vi "VisionExecute.v.vi"(8 "error in (no error)":errorcluster) -> (0 "error out":errorcluster)   [LabVIEW 2023]
uses:
  <vilib>/Rock Robotics/WPI/ThirdParty/PhotonVisionLib/Enum/PhotonPoseStrategy_ENUM.ctl
  <vilib>/Rock Robotics/WPI/ThirdParty/JAS_Junk/TrajLib/TypeDef/POSE2D.ctl
  <vilib>/Rock Robotics/WPI/ThirdParty/JAS_Junk/TrajLib/TypeDef/TRANSLATION2D.ctl
  <vilib>/Rock Robotics/WPI/ThirdParty/JAS_Junk/TrajLib/TypeDef/ROTATION2D.ctl
  <vilib>/Rock Robotics/WPI/ThirdParty/JAS_Junk/TrajLib/VI/AprilTagFieldLayout_New2025.vi
  <vilib>/Rock Robotics/WPI/ThirdParty/JAS_Junk/TrajLib/VI/Util_GetTime_U32.vi
  <vilib>/Rock Robotics/WPI/ThirdParty/PhotonVisionLib/SubVI/PhotonPipelineResult_Unpack.vi
  <vilib>/Rock Robotics/WPI/ThirdParty/PhotonVisionLib/SubVI/PhotonPipelineResult_GetTargetCount.vi
  <vilib>/Rock Robotics/WPI/ThirdParty/PhotonVisionLib/SubVI/PhotonPipelineResult_GetMetadata.vi
  <vilib>/Rock Robotics/WPI/ThirdParty/PhotonVisionLib/SubVI/PhotonPipelineMetadata_GetAll.vi
  <vilib>/Rock Robotics/WPI/ThirdParty/JAS_Junk/TrajLib/VI/Transform3d_Equals.vi
  <vilib>/Rock Robotics/WPI/ThirdParty/PhotonVisionLib/SubVI/PhotonPoseEstimator_SetCamera.vi
  <vilib>/Rock Robotics/WPI/ThirdParty/PhotonVisionLib/SubVI/PhotonPoseEstimator_SetPrimaryStategy.vi
  <vilib>/Rock Robotics/WPI/ThirdParty/PhotonVisionLib/SubVI/PhotonPoseEstimator_SetMultiTagFallbackStrategy.vi
  <vilib>/Rock Robotics/WPI/ThirdParty/PhotonVisionLib/SubVI/PhotonPoseEstimator_SetHighestAmbiguity.vi
  <vilib>/Rock Robotics/WPI/ThirdParty/PhotonVisionLib/SubVI/PhotonPoseEstimator_SetRobotToCameraTransform.vi
  <vilib>/Rock Robotics/WPI/ThirdParty/PhotonVisionLib/SubVI/PhotonPoseEstimator_New.vi
  <vilib>/Rock Robotics/WPI/ThirdParty/PhotonVisionLib/SubVI/PhotonPoseEstimator_SetLastPose.vi
  <vilib>/Rock Robotics/WPI/ThirdParty/PhotonVisionLib/SubVI/PhotonPoseEstimator_Update_PipeResult.vi
  <vilib>/Rock Robotics/WPI/ThirdParty/PhotonVisionLib/SubVI/PhotonPoseEstimator_SetReferencePose.vi
  <vilib>/Rock Robotics/WPI/ThirdParty/PhotonVisionLib/SubVI/PhotonEstimatedRobotPose_GetAll.vi
  <vilib>/Rock Robotics/WPI/ThirdParty/JAS_Junk/TrajLib/VI/Pose3d_ToPose2d.vi
  <vilib>/Rock Robotics/WPI/ThirdParty/JAS_Junk/TrajLib/VI/Quaternion_New.vi
  <vilib>/Rock Robotics/WPI/ThirdParty/JAS_Junk/TrajLib/Conv_Deg_Radians.vi
  <vilib>/Rock Robotics/WPI/ThirdParty/JAS_Junk/TrajLib/VI/TimeInterpDouble_New.vi
  <vilib>/Rock Robotics/WPI/ThirdParty/JAS_Junk/TrajLib/VI/TimeInterpDouble_AddSample.vi
  <vilib>/Rock Robotics/WPI/ThirdParty/JAS_Junk/TrajLib/VI/TimeInterpDouble_GetSample.vi
  <vilib>/Rock Robotics/WPI/ThirdParty/JAS_Junk/TrajLib/VI/TimeInterpDouble_SetMaxTime.vi
  <vilib>/Rock Robotics/WPI/ThirdParty/JAS_Junk/TrajLib/Twist2d_GetAll.vi
  <vilib>/Rock Robotics/WPI/ThirdParty/JAS_Junk/TrajLib/Twist2d_Create.vi
  <vilib>/Rock Robotics/WPI/ThirdParty/JAS_Junk/TrajLib/VI/AprilTagFieldLayout_New.vi
  <vilib>/Rock Robotics/WPI/ThirdParty/JAS_Junk/TrajLib/VI/Pose3d_New_Trans3dRot3d.vi
  <vilib>/Rock Robotics/WPI/ThirdParty/JAS_Junk/TrajLib/VI/Rotation3d_Create_Quaternion.vi
  <vilib>/Rock Robotics/WPI/ThirdParty/JAS_Junk/TrajLib/VI/AprilTag_New.vi
  <vilib>/Rock Robotics/WPI/ThirdParty/JAS_Junk/TrajLib/Timer_New.vi
  <vilib>/Rock Robotics/WPI/ThirdParty/PhotonVisionLib/SubVI/Packet_decode_ByteI8.vi
  <vilib>/Rock Robotics/WPI/ThirdParty/PhotonVisionLib/SubVI/PhotonTrackedTarget_Unpack.vi
  <vilib>/Rock Robotics/WPI/ThirdParty/PhotonVisionLib/SubVI/PhotonMultiTargetPNPResult_unpack.vi
  <vilib>/Rock Robotics/WPI/ThirdParty/PhotonVisionLib/SubVI/PhotonPipelineMetadata_Unpack.vi
  <vilib>/Rock Robotics/WPI/ThirdParty/PhotonVisionLib/SubVI/PhotonPipelineResult_New.vi
  <vilib>/Rock Robotics/WPI/ThirdParty/JAS_Junk/TrajLib/VI/Transform3d_GetTranslation3d.vi
  <vilib>/Rock Robotics/WPI/ThirdParty/JAS_Junk/TrajLib/VI/Transform3d_GetRotation3d.vi
  <vilib>/Rock Robotics/WPI/ThirdParty/JAS_Junk/TrajLib/VI/Rotation3d_Equals.vi
  <vilib>/Rock Robotics/WPI/ThirdParty/JAS_Junk/TrajLib/VI/Translation3d_Equals.vi
  <vilib>/Rock Robotics/WPI/ThirdParty/PhotonVisionLib/SubVI/PhotonTargetModel_New_AprilTag36H11.vi
  <vilib>/Rock Robotics/WPI/ThirdParty/PhotonVisionLib/SubVI/PhotonPoseEstimator_Update_All.vi
  <vilib>/Rock Robotics/WPI/ThirdParty/JAS_Junk/TrajLib/VI/Pose3d_getTranslation3d.vi
  <vilib>/Rock Robotics/WPI/ThirdParty/JAS_Junk/TrajLib/VI/Pose3d_getRotation3d.vi
  <vilib>/Rock Robotics/WPI/ThirdParty/JAS_Junk/TrajLib/VI/Translation3d_ToTranslation2d.vi
  <vilib>/Rock Robotics/WPI/ThirdParty/JAS_Junk/TrajLib/VI/Rotation3d_ToRotation2d.vi
  <vilib>/Rock Robotics/WPI/ThirdParty/JAS_Junk/TrajLib/Pose2d_New_TRRO.vi
  <vilib>/Rock Robotics/WPI/ThirdParty/JAS_Junk/TrajLib/VI/TimeInterpDouble_CleanUp.vi
  <vilib>/Rock Robotics/WPI/ThirdParty/JAS_Junk/TrajLib/MathUtil_Interpolate.vi
  <vilib>/Rock Robotics/WPI/ThirdParty/JAS_Junk/TrajLib/VI/AprilTag_GetAll.vi
  <vilib>/Rock Robotics/WPI/ThirdParty/JAS_Junk/TrajLib/VI/Quaternion_Normalize.vi
  <vilib>/Rock Robotics/WPI/ThirdParty/PhotonVisionLib/SubVI/Packet_decode_Flt64.vi
  <vilib>/Rock Robotics/WPI/ThirdParty/PhotonVisionLib/SubVI/TargetCorner_New.vi
  <vilib>/Rock Robotics/WPI/ThirdParty/PhotonVisionLib/SubVI/Packet_decode_Int32.vi
  <vilib>/Rock Robotics/WPI/ThirdParty/PhotonVisionLib/SubVI/Packet_decode_Transform3d.vi
  <vilib>/Rock Robotics/WPI/ThirdParty/PhotonVisionLib/SubVI/Packet_decode_Flt32.vi
  <vilib>/Rock Robotics/WPI/ThirdParty/PhotonVisionLib/SubVI/Packet_decode_TargetCornerArray.vi
  <vilib>/Rock Robotics/WPI/ThirdParty/PhotonVisionLib/SubVI/Packet_decode_Boolean.vi
  <vilib>/Rock Robotics/WPI/ThirdParty/PhotonVisionLib/SubVI/PhotonPNPResult_unpack.vi
  <vilib>/Rock Robotics/WPI/ThirdParty/PhotonVisionLib/SubVI/PhotonMultiTargetPNPResult_New.vi
  <vilib>/Rock Robotics/WPI/ThirdParty/PhotonVisionLib/SubVI/Packet_decode_Int16.vi
  <vilib>/Rock Robotics/WPI/ThirdParty/PhotonVisionLib/SubVI/Packet_decode_Int64.vi
  <vilib>/Rock Robotics/WPI/ThirdParty/JAS_Junk/TrajLib/VI/Rotation3d_GetQuaterion.vi
  <vilib>/Rock Robotics/WPI/ThirdParty/JAS_Junk/TrajLib/VI/Quaternion_Equals.vi
  <vilib>/Rock Robotics/WPI/ThirdParty/PhotonVisionLib/SubVI/PhotonTargetModel_New_RectPlanar.vi
  <vilib>/Rock Robotics/WPI/ThirdParty/PhotonVisionLib/SubVI/PhotonPoseEstimator_GetEmptyPose.vi
  <vilib>/Rock Robotics/WPI/ThirdParty/PhotonVisionLib/SubVI/PhotonPoseEstimator_lowestAmbiguityStrategy.vi
  <vilib>/Rock Robotics/WPI/ThirdParty/PhotonVisionLib/SubVI/PhotonPoseEstimator_closestToCameraHeightStrategy.vi
  <vilib>/Rock Robotics/WPI/ThirdParty/PhotonVisionLib/SubVI/PhotonPoseEstimator_closestToReferencePoseStrategy.vi
  <vilib>/Rock Robotics/WPI/ThirdParty/PhotonVisionLib/SubVI/PhotonPoseEstimator_GetReferencePose.vi
  <vilib>/Rock Robotics/WPI/ThirdParty/PhotonVisionLib/SubVI/PhotonPoseEstimator_GetLastPose.vi
  <vilib>/Rock Robotics/WPI/ThirdParty/PhotonVisionLib/SubVI/PhotonPoseEstimator_averageBestTargetsStrategy.vi
  <vilib>/Rock Robotics/WPI/ThirdParty/PhotonVisionLib/SubVI/PhotonPoseEstimator_multiTagOnCoprocStrategy.vi
  <vilib>/Rock Robotics/WPI/ThirdParty/PhotonVisionLib/SubVI/PhotonPipelineResult_GetTimeStampSecs.vi
  <vilib>/Rock Robotics/WPI/ThirdParty/JAS_Junk/TrajLib/Translation2d_Create.vi
  <vilib>/Rock Robotics/WPI/ThirdParty/JAS_Junk/TrajLib/Rotation2d_CreateAngle.vi
  <vilib>/Rock Robotics/WPI/ThirdParty/JAS_Junk/TrajLib/VI/Rotation3d_GetXYZ.vi
  <vilib>/Rock Robotics/WPI/ThirdParty/JAS_Junk/TrajLib/MathUtil_Clamp.vi
  <vilib>/Rock Robotics/WPI/ThirdParty/JAS_Junk/TrajLib/VI/Quaternion_New_Default.vi
  <vilib>/Rock Robotics/WPI/ThirdParty/PhotonVisionLib/SubVI/PhotonPNPResult_New.vi
  <vilib>/Rock Robotics/WPI/ThirdParty/JAS_Junk/TrajLib/VI/Quaternion_Get_Vect.vi
  <vilib>/Rock Robotics/WPI/ThirdParty/JAS_Junk/TrajLib/VI/Quaternion_Get_W.vi
  <vilib>/Rock Robotics/WPI/ThirdParty/PhotonVisionLib/SubVI/PhotonTargetModel_New.vi
  <vilib>/Rock Robotics/WPI/ThirdParty/JAS_Junk/TrajLib/VI/Rotation3d_Create_AxisAngle.vi
  <vilib>/Rock Robotics/WPI/ThirdParty/JAS_Junk/TrajLib/VI/Pose3d_New.vi
  <vilib>/Rock Robotics/WPI/ThirdParty/PhotonVisionLib/SubVI/PhotonPipelineResult_HasTargets.vi
  <vilib>/Rock Robotics/WPI/ThirdParty/PhotonVisionLib/SubVI/PhotonPipelineResult_GetTargets.vi
  <vilib>/Rock Robotics/WPI/ThirdParty/PhotonVisionLib/SubVI/PhotonTrackedTarget_GetPoseAmbiguity.vi
  <vilib>/Rock Robotics/WPI/ThirdParty/PhotonVisionLib/SubVI/PhotonTrackedTarget_GetFiducialId.vi
  <vilib>/Rock Robotics/WPI/ThirdParty/PhotonVisionLib/SubVI/PhotonPoseEstimator_GetFieldTags.vi
  <vilib>/Rock Robotics/WPI/ThirdParty/JAS_Junk/TrajLib/VI/AprilTagFieldLayout_GetTagPose.vi
  <vilib>/Rock Robotics/WPI/ThirdParty/JAS_Junk/TrajLib/VI/Pose3d_TransformBy.vi
  <vilib>/Rock Robotics/WPI/ThirdParty/PhotonVisionLib/SubVI/PhotonTrackedTarget_GetBestCameraToTarget.vi
  <vilib>/Rock Robotics/WPI/ThirdParty/JAS_Junk/TrajLib/VI/Transform3d_Inverse.vi
  <vilib>/Rock Robotics/WPI/ThirdParty/PhotonVisionLib/SubVI/PhotonPoseEstimator_GetRobotToCameraTransform.vi
  <vilib>/Rock Robotics/WPI/ThirdParty/PhotonVisionLib/SubVI/PhotonPoseEstimator_GetHighestAmbiguity.vi
  <vilib>/Rock Robotics/WPI/ThirdParty/PhotonVisionLib/SubVI/PhotonEstimatedRobotPose_New.vi
  <vilib>/Rock Robotics/WPI/ThirdParty/PhotonVisionLib/SubVI/PhotonPoseEstimator_closestToCameraHeightStrategy_calc.vi
  <vilib>/Rock Robotics/WPI/ThirdParty/PhotonVisionLib/SubVI/PhotonTrackedTarget_GetAltCameraToTarget.vi
  <vilib>/Rock Robotics/WPI/ThirdParty/PhotonVisionLib/SubVI/PhotonPoseEstimator_closestToReferencePoseStrategy_calc.vi
  <vilib>/Rock Robotics/WPI/ThirdParty/PhotonVisionLib/SubVI/PhotonPoseEstimator_averageBestTargetsStrategy_calc.vi
  <vilib>/Rock Robotics/WPI/ThirdParty/JAS_Junk/TrajLib/VI/Rotation3d_Plus.vi
  <vilib>/Rock Robotics/WPI/ThirdParty/JAS_Junk/TrajLib/VI/Translation3d_Plus.vi
  <vilib>/Rock Robotics/WPI/ThirdParty/JAS_Junk/TrajLib/VI/Translation3d_Times.vi
  <vilib>/Rock Robotics/WPI/ThirdParty/JAS_Junk/TrajLib/VI/Rotation3d_Times.vi
  <vilib>/Rock Robotics/WPI/ThirdParty/JAS_Junk/TrajLib/VI/Rotation3d_Create_Default.vi
  <vilib>/Rock Robotics/WPI/ThirdParty/JAS_Junk/TrajLib/VI/Translation3d_Create_Default.vi
  <vilib>/Rock Robotics/WPI/ThirdParty/JAS_Junk/TrajLib/VI/Pose3d_New_Default.vi
  <vilib>/Rock Robotics/WPI/ThirdParty/JAS_Junk/TrajLib/VI/Pose3d_Plus.vi
  <vilib>/Rock Robotics/WPI/ThirdParty/JAS_Junk/TrajLib/VI/Pose3d_RelativeTo.vi
  <vilib>/Rock Robotics/WPI/ThirdParty/JAS_Junk/TrajLib/VI/AprilTagFieldLayout_GetOriginPosition.vi
  <vilib>/Rock Robotics/WPI/ThirdParty/PhotonVisionLib/SubVI/PhotonPipelineResult_GetMultiTagResult.vi
  <vilib>/Rock Robotics/WPI/ThirdParty/JAS_Junk/TrajLib/VI/Quaternion_Get_All.vi
  <vilib>/Rock Robotics/WPI/ThirdParty/JAS_Junk/TrajLib/VI/Vector_Norm.vi
  <vilib>/Rock Robotics/WPI/ThirdParty/JAS_Junk/TrajLib/VecBuilder_ArrayBy1Fill.vi
  <vilib>/Rock Robotics/WPI/ThirdParty/JAS_Junk/TrajLib/VI/Translation3d_RotateBy.vi
  <vilib>/Rock Robotics/WPI/ThirdParty/JAS_Junk/TrajLib/Transform2d_Create_TransRot.vi
  <vilib>/Rock Robotics/WPI/ThirdParty/JAS_Junk/TrajLib/VI/Rotation3d_UnaryMinus.vi
  <vilib>/Rock Robotics/WPI/ThirdParty/JAS_Junk/TrajLib/VI/Translation3d_UnaryMinus.vi
  <vilib>/Rock Robotics/WPI/ThirdParty/JAS_Junk/TrajLib/VI/Transform3d_GetXYZ.vi
  <vilib>/Rock Robotics/WPI/ThirdParty/JAS_Junk/TrajLib/VI/Pose3d_getXYZ.vi
  <vilib>/Rock Robotics/WPI/ThirdParty/PhotonVisionLib/SubVI/PhotonPoseEstimator_CalcDifference.vi
  <vilib>/Rock Robotics/WPI/ThirdParty/JAS_Junk/TrajLib/VI/Rotation3d_RotateBy.vi
  <vilib>/Rock Robotics/WPI/ThirdParty/JAS_Junk/TrajLib/VI/Translation3d_GetXYZ.vi
  <vilib>/Rock Robotics/WPI/ThirdParty/JAS_Junk/TrajLib/VI/Transform3d_Create_Pose3dPose3d.vi
  <vilib>/Rock Robotics/WPI/ThirdParty/JAS_Junk/TrajLib/MatBuilder_Create.vi
  <vilib>/Rock Robotics/WPI/ThirdParty/JAS_Junk/TrajLib/VI/Quaternion_Times.vi
  <vilib>/Rock Robotics/WPI/ThirdParty/JAS_Junk/TrajLib/VI/Quaternion_Inverse.vi
  <vilib>/Rock Robotics/WPI/ThirdParty/JAS_Junk/TrajLib/VI/Translation3d_GetDistance.vi
  <vilib>/Rock Robotics/WPI/ThirdParty/JAS_Junk/TrajLib/VI/Translation3d_Minus.vi
  <vilib>/Rock Robotics/WPI/ThirdParty/JAS_Junk/TrajLib/VI/Rotation3d_Minus.vi
  Robot Global Data.vi
  VisionGlobal.vi
  <vilib>/Rock Robotics/SystemInterfaces/Utilities/FPGA_UtilitiesRead LocalTime.vi
  <vilib>/Rock Robotics/WPI/ThirdParty/JAS_Junk/TrajLib/VI/Util_GetTime_U64.vi
  <vilib>/Rock Robotics/Network Tables/NT Read Value.vi
  <vilib>/Rock Robotics/Network Tables/NT Read Raw.vi
  <vilib>/Utility/semaphor.llb/Obtain Semaphore Reference.vi
  <vilib>/Rock Robotics/WPI/ThirdParty/JAS_Junk/TrajLib/Timer_Reset.vi
  <vilib>/Rock Robotics/WPI/ThirdParty/JAS_Junk/TrajLib/Timer_Start.vi
  <vilib>/Rock Robotics/WPI/ThirdParty/JAS_Junk/TrajLib/Timer_Stop.vi
  <vilib>/Rock Robotics/WPI/ThirdParty/JAS_Junk/TrajLib/Timer_HasPeriodPassedOnce.vi
  <vilib>/gmath/interp.llb/Search Ordered Table.vi
  <vilib>/Rock Robotics/WPI/ThirdParty/JAS_Junk/TrajLib/Pose2d_Log.vi
  <vilib>/Rock Robotics/WPI/ThirdParty/JAS_Junk/TrajLib/Pose2d_Exp.vi
  <vilib>/Rock Robotics/WPI/ThirdParty/JAS_Junk/TrajLib/Trajectory_Library.lvlib
  <vilib>/Rock Robotics/WPI/ThirdParty/PhotonVisionLib/PhotonVisionLib.lvlib
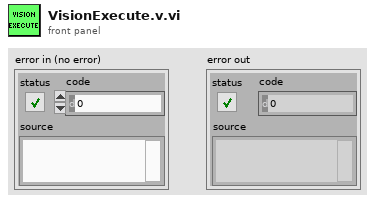
[diagram p1: front panel]
types:
  T1 = typedef "PhotonVisionLib.lvlib/PhotonPoseStrategy_ENUM.ctl" = enum16{"LOWEST_AMBIGUITY", "CLOSEST_TO_CAMERA_HEIGHT", "CLOSEST_TO_REFERENCE_POSE", "CLOSEST_TO_LAST_POSE", "AVERAGE_BEST_TARGETS", "MULTI_TAG_PNP_ON_COPROCESSOR", "MULTI_TAG_PNP_ON_RIO"}
  T2 = typedef "Trajectory_Library.lvlib/TRANSLATION3D.ctl" = cluster{"X":dbl, "Y":dbl, "Z":dbl}
  T3 = typedef "Trajectory_Library.lvlib/ROTATION3D.ctl" = cluster{"Q_quaternion":T4}
  T4 = typedef "Trajectory_Library.lvlib/QUATERNION.ctl" = cluster{"R":dbl, "V":dbl[]}
  T5 = typedef "Trajectory_Library.lvlib/TRANSFORM3D.ctl" = cluster{"TRANSLATION3D":T2, "ROTATION3D":T3, "XF":bool}
  T6 = typedef "PhotonVisionLib.lvlib/PhotonPipelineResultType.ctl" = cluster{"Targets":T7[], "PhotonMultiTargetPNPResult":T9, "PhotonPipelineMetadata":T11}
  T7 = typedef "PhotonVisionLib.lvlib/PhotonTrackedTargetType.ctl" = cluster{"Yaw":dbl, "Pitch":dbl, "Area":dbl, "Skew":dbl, "MinAreaRectCorners":T8[], "BestCameraToTarget":T5, "FiducialId":i32, "AltCameraToTarget":T5, "PoseAmbiguity":dbl, "DetectedCorners":T8[], "ObjDetectId":i32, "ObjDetectConf":sgl}
  T8 = typedef "PhotonVisionLib.lvlib/TargetCornerType.ctl" = cluster{"X":dbl, "Y":dbl}
  T9 = typedef "PhotonVisionLib.lvlib/PhotonMultiTargetPNPResultType.ctl" = cluster{"PhotonPNPResult":T10, "FiducialIDsUsed":i16[]}
  T10 = typedef "PhotonVisionLib.lvlib/PhotonPNPResultType.ctl" = cluster{"IsPresent":bool, "bestReprojErr":dbl, "altReprojErr":dbl, "ambiguity":dbl, "Best":T5, "Alt":T5}
  T11 = typedef "PhotonVisionLib.lvlib/PhotonPipelineMetadataType.ctl" = cluster{"CaptureTimestampMicros":i64, "PublishTimestampMicros":i64, "SequenceID":i64, "TimeSinceLastPong":i64}
  T12 = typedef "Trajectory_Library.lvlib/AprilTagFieldLayout.ctl" = cluster{"AprilTagMap":map{i32, T13}, "FieldLength":dbl, "FieldWidth":dbl, "OriginPosition ":T15, "OriginPose3d":T14}
  T13 = typedef "Trajectory_Library.lvlib/AprilTag.ctl" = cluster{"ID":i32, "POSE3D":T14}
  T14 = typedef "Trajectory_Library.lvlib/POSE3D.ctl" = cluster{"Translation3d":T2, "Rotation3d":T3}
  T15 = typedef "Trajectory_Library.lvlib/AprilTagFieldLayoutOrignPosition_ENUM.ctl" = enum16{"kBlueAllianceWallRightSide,", "kRedAllianceWallRightSide,"}
  T16 = typedef "PhotonVisionLib.lvlib/PhotonPoseEstimator_Configuration.ctl" = cluster{"Primary Strategy":T1, "Camera":string, "Initial Pose":T14, "HighestAmbiguity":dbl, "RobotToCamera":T5, "FallBack Strategy":T1, "BaseNTName":string}
  T17 = typedef "Trajectory_Library.lvlib/POSE2D.ctl" = cluster{"TRANSLATION":T18, "ROTATION":T19}
  T18 = typedef "Trajectory_Library.lvlib/TRANSLATION2D.ctl" = cluster{"X":dbl, "Y":dbl}
  T19 = typedef "Trajectory_Library.lvlib/ROTATION2D.ctl" = cluster{"VALUE":dbl, "COS":dbl, "SIN":dbl}
  T20 = typedef "Trajectory_Library.lvlib/SWERVE_DRIVE_KINEMATICS.ctl" = cluster{"NumModules":i32, "InverseKinematics":T21, "ForwardKinematics":T21, "Modules":T18[], "PrevCoR":T18, "SavedModuleStates":T22[]}
  T21 = typedef "NI_Matrix.lvlib/RealMatrix.ctl" = dbl[][]
  T22 = typedef "Trajectory_Library.lvlib/SWERVE_DRIVE_MODULE_STATE.ctl" = cluster{"Speed":dbl, "Angle":T19}
  T23 = typedef "Trajectory_Library.lvlib/SWERVE_DRIVE_MODULE_POSITION.ctl" = cluster{"Distance":dbl, "Angle":T19, "P":bool}
  T24 = typedef "Trajectory_Library.lvlib/SWERVE_DRIVE_POSE_EST2_CONFIG.ctl" = cluster{"Wheel_Locations M":T18[], "Odom X std dev M":dbl, "Odom Y std dev M":dbl, "Odom Heading std dev Rad":dbl, "Vision X std dev M":dbl, "Vision Y std dev M":dbl, "Vision Heading std dev Rad":dbl}
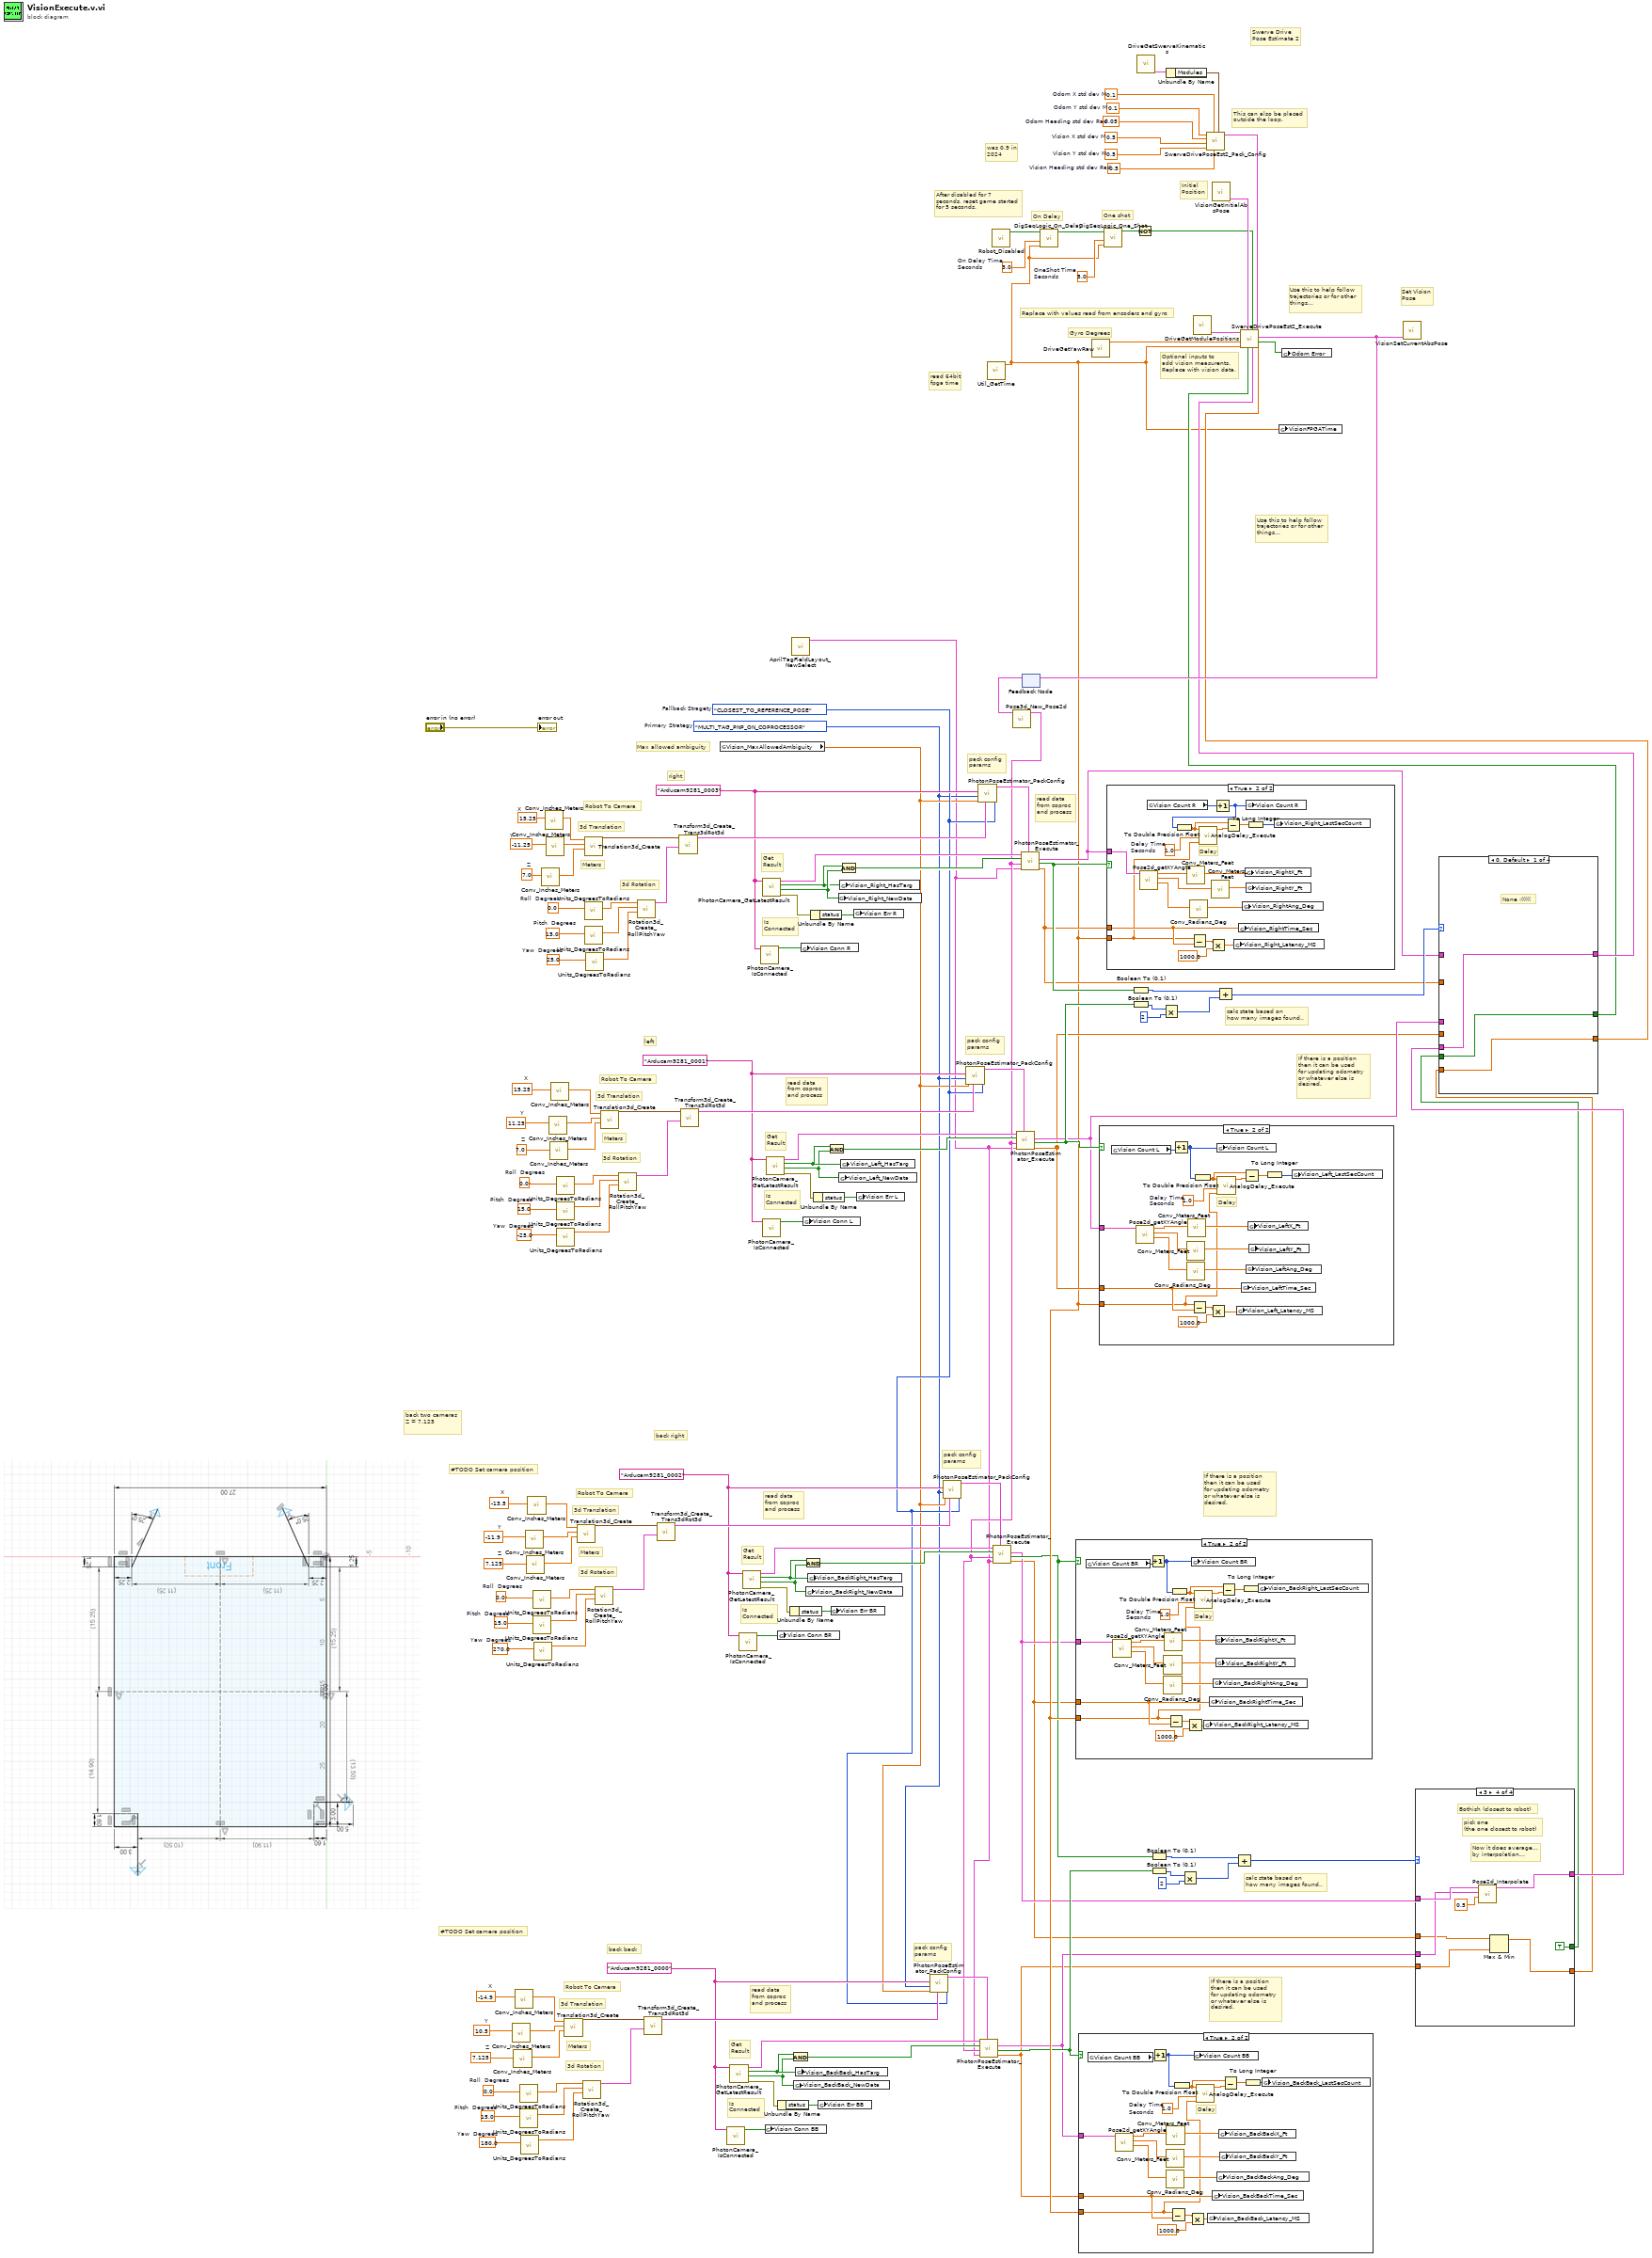
[diagram p0: block diagram]
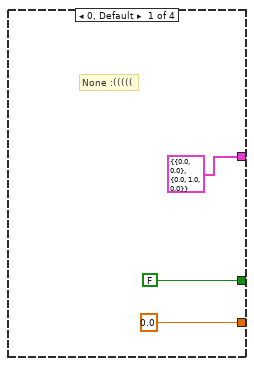
[diagram p2: hidden frame]
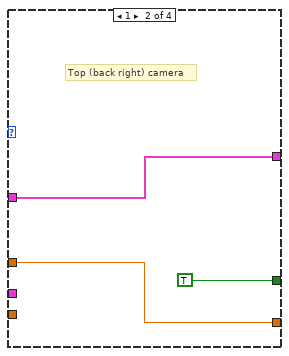
[diagram p3: hidden frame]
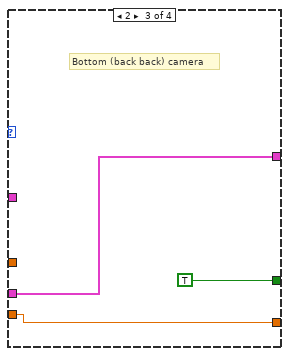
[diagram p4: hidden frame]
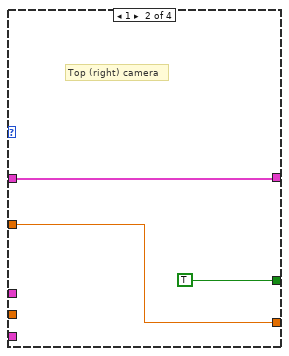
[diagram p7: hidden frame]
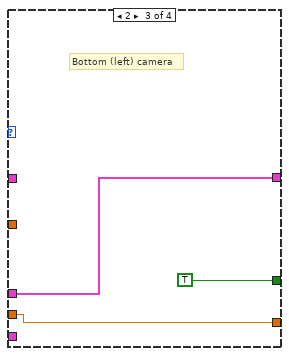
[diagram p8: hidden frame]
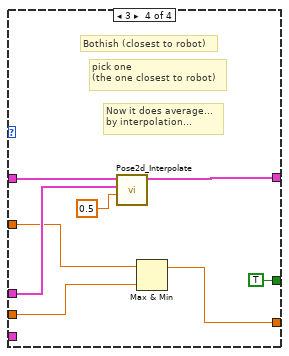
[diagram p9: hidden frame]
diagram:
  w39 = 0.0  # Roll  Degrees
  w38 = 15.0  # Pitch  Degrees
  w37 = 180.0  # Yaw  Degrees
  w24 = 7.125  # Z
  w28 = -14.9  # X
  w26 = 10.5  # Y
  w33 = "Arducam9281_0000" ("CameraName")
  w63 = 0.0  # Roll  Degrees
  w62 = 15.0  # Pitch  Degrees
  w61 = 270.0  # Yaw  Degrees
  w48 = 7.125  # Z
  w52 = -13.5  # X
  w50 = -11.9  # Y
  w57 = "Arducam9281_0002" ("CameraName")
  w78 = 5.0  # OneShot Time Seconds
  w80 = 3.0  # On Delay Time Seconds
  w20 = PhotonPoseStrategy_ENUM."CLOSEST_TO_REFERENCE_POSE"  # Fallback Stragety
  w96 = 0.1  # Odom Y std dev M
  w97 = 0.05  # Odom Heading std dev Rad
  w98 = 0.5  # Vision X std dev M
  w99 = 0.5  # Vision Y std dev M
  w100 = 0.1  # Odom X std dev M
  w101 = 0.5  # Vision Heading std dev Rad
  w131 = 0.0  # Roll  Degrees
  w130 = 15.0  # Pitch  Degrees
  w129 = -25.0  # Yaw  Degrees
  w116 = 7.0  # Z
  w120 = 15.25  # X
  w118 = 11.25  # Y
  w125 = "Arducam9281_0001" ("CameraName")
  w147 = 0.0  # Roll  Degrees
  w146 = 15.0  # Pitch  Degrees
  w145 = 25.0  # Yaw  Degrees
  w110 = 7.0  # Z
  w114 = 15.25  # X
  w112 = -11.25  # Y
  w18 = PhotonPoseStrategy_ENUM."MULTI_TAG_PNP_ON_COPROCESSOR"  # Primary Strategy
  w141 = "Arducam9281_0003" ("CameraName")
  # "calc state based on\nhow many images found.."
  # "#TODO Set camera position"
  # "#TODO Set camera position"
  # "back right"
  # "read data\nfrom coproc\nand process"
  # "pack config\nparams"
  # "back back"
  # "Meters"
  # "Robot To Camera"
  # "3d Rotation"
  # "3d Translation"
  # "Is\nConnected"
  # "Get\nResult"
  # "If there is a position\nthen it can be used\nfor updating odometry\nor whatever else is \ndesired."
  # "read data\nfrom coproc\nand process"
  # "pack config\nparams"
  # "Meters"
  # "Robot To Camera"
  # "3d Rotation"
  # "3d Translation"
  # "Is\nConnected"
  # "Get\nResult"
  # "If there is a position\nthen it can be used\nfor updating odometry\nor whatever else is \ndesired."
  # "Max allowed ambiguity"
  # "back two cameras\nZ = 7.125"
  # "Set Vision\nPose"
  # "After disabled for 7\nseconds, reset game started\nfor 5 seconds."
  # "One shot"
  # "On Delay"
  # "was 0.9 in\n2024"
  # "calc state based on\nhow many images found.."
  # "read data\nfrom coproc\nand process"
  # "read data\nfrom coproc\nand process"
  # "pack config\nparams"
  # "pack config\nparams"
  # "Initial\nPosition"
  # "Optional inputs to\nadd vision measurents.\nReplace with vision data."
  # "Replace with values read from encoders and gyro"
  # "read 64bit\nfpga time"
  # "This can also be placed \noutside the loop."
  # "Use this to help follow\ntrajectories or for other\nthings..."
  # "Swerve Drive \nPose Estimate 2"
  # "Use this to help follow\ntrajectories or for other\nthings..."
  # "right"
  # "left"
  # "Meters"
  # "Robot To Camera"
  # "3d Rotation"
  # "3d Translation"
  # "Is\nConnected"
  # "Get\nResult"
  # "If there is a position\nthen it can be used\nfor updating odometry\nor whatever else is \ndesired."
  # "Meters"
  # "Robot To Camera"
  # "3d Rotation"
  # "3d Translation"
  # "Is\nConnected"
  # "Get\nResult"
  # "Gyro Degrees"
  n1 = call <vilib>:"Conv_Inches_Meters.vi"("INCH"=w26) -> ("Meters"=w25:dbl)  [unwired: 10 in]
  n2 = call <vilib>:"Conv_Inches_Meters.vi"("INCH"=w24) -> ("Meters"=w23:dbl)  [unwired: 10 in]
  n3 = call <vilib>:"Conv_Inches_Meters.vi"("INCH"=w28) -> ("Meters"=w27:dbl)  [unwired: 10 in]
  n4 = call <vilib>:"Units_DegreesToRadians.vi"("Degrees"=w39) -> ("Radians"=w36:dbl)  [unwired: 10 in]
  n5 = call <vilib>:"Units_DegreesToRadians.vi"("Degrees"=w38) -> ("Radians"=w35:dbl)  [unwired: 10 in]
  n6 = call <vilib>:"Units_DegreesToRadians.vi"("Degrees"=w37) -> ("Radians"=w34:dbl)  [unwired: 10 in]
  n7 = call <vilib>:"Conv_Inches_Meters.vi"("INCH"=w50) -> ("Meters"=w49:dbl)  [unwired: 10 in]
  n8 = call <vilib>:"Conv_Inches_Meters.vi"("INCH"=w48) -> ("Meters"=w47:dbl)  [unwired: 10 in]
  n9 = call <vilib>:"Conv_Inches_Meters.vi"("INCH"=w52) -> ("Meters"=w51:dbl)  [unwired: 10 in]
  n10 = call <vilib>:"Units_DegreesToRadians.vi"("Degrees"=w63) -> ("Radians"=w60:dbl)  [unwired: 10 in]
  n11 = call <vilib>:"Units_DegreesToRadians.vi"("Degrees"=w62) -> ("Radians"=w59:dbl)  [unwired: 10 in]
  n12 = call <vilib>:"Units_DegreesToRadians.vi"("Degrees"=w61) -> ("Radians"=w58:dbl)  [unwired: 10 in]
  n13 = call <vilib>:"Conv_Inches_Meters.vi"("INCH"=w110) -> ("Meters"=w109:dbl)  [unwired: 10 in]
  n14 = call <vilib>:"Conv_Inches_Meters.vi"("INCH"=w114) -> ("Meters"=w113:dbl)  [unwired: 10 in]
  n15 = call <vilib>:"Conv_Inches_Meters.vi"("INCH"=w112) -> ("Meters"=w111:dbl)  [unwired: 10 in]
  n16 = call <vilib>:"Conv_Inches_Meters.vi"("INCH"=w118) -> ("Meters"=w117:dbl)  [unwired: 10 in]
  n17 = call <vilib>:"Conv_Inches_Meters.vi"("INCH"=w116) -> ("Meters"=w115:dbl)  [unwired: 10 in]
  n18 = call <vilib>:"Conv_Inches_Meters.vi"("INCH"=w120) -> ("Meters"=w119:dbl)  [unwired: 10 in]
  n19 = call <vilib>:"Units_DegreesToRadians.vi"("Degrees"=w131) -> ("Radians"=w128:dbl)  [unwired: 10 in]
  n20 = call <vilib>:"Units_DegreesToRadians.vi"("Degrees"=w130) -> ("Radians"=w127:dbl)  [unwired: 10 in]
  n21 = call <vilib>:"Units_DegreesToRadians.vi"("Degrees"=w129) -> ("Radians"=w126:dbl)  [unwired: 10 in]
  n22 = call <vilib>:"Translation3d_Create.vi"("Z"=w23, "Y"=w25, "X"=w27) -> ("TRANSLATION3D"=w40:T2)  [unwired: 8 in]
  n23 = call <vilib>:"Translation3d_Create.vi"("Z"=w47, "Y"=w49, "X"=w51) -> ("TRANSLATION3D"=w64:T2)  [unwired: 8 in]
  n24 = call <vilib>:"Rotation3d_Create_RollPitchYaw.vi"("Yaw"=w34, "Pitch"=w35, "Roll"=w36) -> ("Rotation3d"=w41:T3)  [unwired: 8 in]
  n25 = call <vilib>:"Translation3d_Create.vi"("Z"=w109, "Y"=w111, "X"=w113) -> ("TRANSLATION3D"=w148:T2)  [unwired: 8 in]
  n26 = call <vilib>:"Units_DegreesToRadians.vi"("Degrees"=w147) -> ("Radians"=w144:dbl)  [unwired: 10 in]
  n27 = call <vilib>:"Units_DegreesToRadians.vi"("Degrees"=w146) -> ("Radians"=w143:dbl)  [unwired: 10 in]
  n28 = call <vilib>:"Units_DegreesToRadians.vi"("Degrees"=w145) -> ("Radians"=w142:dbl)  [unwired: 10 in]
  n29 = call <vilib>:"Rotation3d_Create_RollPitchYaw.vi"("Yaw"=w58, "Pitch"=w59, "Roll"=w60) -> ("Rotation3d"=w65:T3)  [unwired: 8 in]
  n30 = call <vilib>:"Translation3d_Create.vi"("Z"=w115, "Y"=w117, "X"=w119) -> ("TRANSLATION3D"=w132:T2)  [unwired: 8 in]
  n31 = call <vilib>:"Rotation3d_Create_RollPitchYaw.vi"("Yaw"=w126, "Pitch"=w127, "Roll"=w128) -> ("Rotation3d"=w133:T3)  [unwired: 8 in]
  n32 = call <vilib>:"Rotation3d_Create_RollPitchYaw.vi"("Yaw"=w142, "Pitch"=w143, "Roll"=w144) -> ("Rotation3d"=w149:T3)  [unwired: 8 in]
  n33 = call <vilib>:"Transform3d_Create_Trans3dRot3d.vi"("Rotation3d"=w41, "Translation3d"=w40) -> ("Transform3d"=w42:T5)  [unwired: 9 in]
  n34 = call <vilib>:"Transform3d_Create_Trans3dRot3d.vi"("Rotation3d"=w65, "Translation3d"=w64) -> ("Transform3d"=w66:T5)  [unwired: 9 in]
  n35 = call <vilib>:"Transform3d_Create_Trans3dRot3d.vi"("Rotation3d"=w149, "Translation3d"=w148) -> ("Transform3d"=w150:T5)  [unwired: 9 in]
  n36 = call <vilib>:"Transform3d_Create_Trans3dRot3d.vi"("Rotation3d"=w133, "Translation3d"=w132) -> ("Transform3d"=w134:T5)  [unwired: 9 in]
  n37 = global read "VisionGlobal.vi" "Vision_MaxAllowedAmbiguity"() -> (w19:dbl)
  n38 = call <vilib>:"PhotonCamera_IsConnected.vi"("CameraName"=w33) -> ("IsConnected"=w31:bool)  [unwired: 9 in, 1 out]
  n39 = call <vilib>:"PhotonCamera_GetLatestResult.vi"("CameraName"=w33) -> ("error out"=w30:errorcluster, "New Data"=w21:bool, "HasTargets"=w22:bool, "PipelineResult"=w43:T6)  [unwired: 6 in, 1 out]
  n40 = call <vilib>:"PhotonCamera_IsConnected.vi"("CameraName"=w57) -> ("IsConnected"=w55:bool)  [unwired: 9 in, 1 out]
  n41 = call <vilib>:"PhotonCamera_GetLatestResult.vi"("CameraName"=w57) -> ("error out"=w54:errorcluster, "New Data"=w45:bool, "HasTargets"=w46:bool, "PipelineResult"=w67:T6)  [unwired: 6 in, 1 out]
  n42 = call <vilib>:"PhotonCamera_IsConnected.vi"("CameraName"=w141) -> ("IsConnected"=w139:bool)  [unwired: 9 in, 1 out]
  n43 = call <vilib>:"PhotonCamera_GetLatestResult.vi"("CameraName"=w141) -> ("error out"=w138:errorcluster, "New Data"=w73:bool, "HasTargets"=w72:bool, "PipelineResult"=w151:T6)  [unwired: 6 in, 1 out]
  n44 = call <vilib>:"PhotonCamera_IsConnected.vi"("CameraName"=w125) -> ("IsConnected"=w123:bool)  [unwired: 9 in, 1 out]
  n45 = global write "VisionGlobal.vi" "Vision Conn BB"(w31) -> ()
  n46 = call <vilib>:"PhotonCamera_GetLatestResult.vi"("CameraName"=w125) -> ("error out"=w122:errorcluster, "New Data"=w70:bool, "HasTargets"=w71:bool, "PipelineResult"=w135:T6)  [unwired: 6 in, 1 out]
  n47 = Unbundle By Name(w30) -> ("status"=w29:bool)
  n48 = global write "VisionGlobal.vi" "Vision Conn BR"(w55) -> ()
  n49 = Unbundle By Name(w54) -> ("status"=w53:bool)
  n50 = call-poly <vilib>:"AprilTagFieldLayout_NewSelect.vi"() -> ("AprilTagFieldLayout"=w16:T12)  [unwired: 11 in]
  n51 = And(x=w22, y=w21) -> (x .and. y?=w44:bool)
  n52 = global write "VisionGlobal.vi" "Vision_BackBack_NewData"(w21) -> ()
  n53 = global write "VisionGlobal.vi" "Vision_BackBack_HasTarg"(w22) -> ()
  n54 = global write "VisionGlobal.vi" "Vision Conn R"(w139) -> ()
  n55 = global write "VisionGlobal.vi" "Vision Conn L"(w123) -> ()
  n56 = And(x=w46, y=w45) -> (x .and. y?=w68:bool)
  n57 = global write "VisionGlobal.vi" "Vision_BackRight_NewData"(w45) -> ()
  n58 = global write "VisionGlobal.vi" "Vision_BackRight_HasTarg"(w46) -> ()
  n59 = Unbundle By Name(w138) -> ("status"=w137:bool)
  n60 = Unbundle By Name(w122) -> ("status"=w121:bool)
  n61 = global write "VisionGlobal.vi" "Vision Err BB"(w29) -> ()
  n62 = And(x=w71, y=w70) -> (x .and. y?=w136:bool)
  n63 = global write "VisionGlobal.vi" "Vision Err BR"(w53) -> ()
  n64 = global write "VisionGlobal.vi" "Vision_Right_NewData"(w73) -> ()
  n65 = global write "VisionGlobal.vi" "Vision_Left_NewData"(w70) -> ()
  n66 = And(x=w72, y=w73) -> (x .and. y?=w152:bool)
  n67 = global write "VisionGlobal.vi" "Vision_Right_HasTarg"(w72) -> ()
  n68 = global write "VisionGlobal.vi" "Vision_Left_HasTarg"(w71) -> ()
  n69 = global write "VisionGlobal.vi" "Vision Err R"(w137) -> ()
  n70 = global write "VisionGlobal.vi" "Vision Err L"(w121) -> ()
  n71 = call <vilib>:"PhotonPoseEstimator_PackConfig.vi"("FallBack Strategy"=w20, "RobotToCamera"=w42, "HighestAmbiguity"=w19, "PirmaryStrategy"=w18, "Camera"=w33) -> ("PoseEstimator_Configuration"=w32:T16)  [unwired: 6 in]
  n72 = call <vilib>:"PhotonPoseEstimator_PackConfig.vi"("FallBack Strategy"=w20, "RobotToCamera"=w66, "HighestAmbiguity"=w19, "PirmaryStrategy"=w18, "Camera"=w57) -> ("PoseEstimator_Configuration"=w56:T16)  [unwired: 6 in]
  n73 = call <vilib>:"PhotonPoseEstimator_PackConfig.vi"("FallBack Strategy"=w20, "RobotToCamera"=w134, "HighestAmbiguity"=w19, "PirmaryStrategy"=w18, "Camera"=w125) -> ("PoseEstimator_Configuration"=w124:T16)  [unwired: 6 in]
  n74 = call <vilib>:"PhotonPoseEstimator_PackConfig.vi"("FallBack Strategy"=w20, "RobotToCamera"=w150, "HighestAmbiguity"=w19, "PirmaryStrategy"=w18, "Camera"=w141) -> ("PoseEstimator_Configuration"=w140:T16)  [unwired: 6 in]
  n75 = call <vilib>:"Util_GetTime.vi"() -> ("FPGA_Time_Seconds"=w15:dbl)  [unwired: 9 in, 2 out]
  n76 = call "Robot_Disabled.vi"() -> ("Robot Disabled"=w79:bool)  [unwired: 11 in]
  n77 = feedback #1() -> (w74:T17)  [unwired: 1 in]
  n78 = call <vilib>:"Pose3d_New_Pose2d.vi"("in POSE2D"=w74) -> ("out Pose3d"=w17:T14)  [unwired: 10 in]
  n79 = call <vilib>:"PhotonPoseEstimator_Execute.vi"("Configuration"=w32, "AprilTagFieldLayout"=w16, "ReferencePose"=w17, "PIpeline Has \nNew Results"=w44, "PipelineResult"=w43) -> ("TimeStamp_Seconds"=w4:dbl, "New Pose Found"=w9:bool, "EstimatedPose2d"=w6:T17)  [unwired: 4 out]
  n80 = call <vilib>:"PhotonPoseEstimator_Execute.vi"("Configuration"=w56, "AprilTagFieldLayout"=w16, "ReferencePose"=w17, "PIpeline Has \nNew Results"=w68, "PipelineResult"=w67) -> ("TimeStamp_Seconds"=w5:dbl, "New Pose Found"=w10:bool, "EstimatedPose2d"=w7:T17)  [unwired: 4 out]
  n81 = call <vilib>:"PhotonPoseEstimator_Execute.vi"("Configuration"=w124, "AprilTagFieldLayout"=w16, "ReferencePose"=w17, "PIpeline Has \nNew Results"=w136, "PipelineResult"=w135) -> ("TimeStamp_Seconds"=w84:dbl, "New Pose Found"=w107:bool, "EstimatedPose2d"=w86:T17)  [unwired: 4 out]
  n82 = call <vilib>:"PhotonPoseEstimator_Execute.vi"("Configuration"=w140, "AprilTagFieldLayout"=w16, "ReferencePose"=w17, "PIpeline Has \nNew Results"=w152, "PipelineResult"=w151) -> ("TimeStamp_Seconds"=w83:dbl, "New Pose Found"=w108:bool, "EstimatedPose2d"=w85:T17)  [unwired: 4 out]
  n83 = call <vilib>:"DigSeqLogic_On_Delay.vi"("Time"=w15, "Delay"=w80, "Input"=w79) -> ("Output"=w77:bool)  [unwired: 7 in, 1 out]
  n84 = case shown="True" w10 {
    tunnel: w7 -> [_ w170]
    tunnel: w5 -> [_ w160]
    tunnel: w15 -> [_ w153]
    frame False {
    }
    frame True {
      w159 = 1.0  # Delay Time Seconds
      # "Delay"
      n85 = global read "VisionGlobal.vi" "Vision Count BR"() -> (w171:i32)
      n86 = call <vilib>:"Pose2d_getXYAngle.vi"("in POSE"=w170) -> ("Angle"=w167:dbl, "Y"=w168:dbl, "X"=w169:dbl)  [unwired: 8 in]
      n87 = Increment(x=w171) -> (x+1=w158:i32)
      n88 = call <vilib>:"Conv_Meters_Feet.vi"("Meters"=w168) -> ("Feet"=w165:dbl)  [unwired: 10 in]
      n89 = call <vilib>:"Conv_Radians_Deg.vi"("Radians"=w167) -> ("Degrees"=w164:dbl)  [unwired: 10 in]
      n90 = call <vilib>:"Conv_Meters_Feet.vi"("Meters"=w169) -> ("Feet"=w166:dbl)  [unwired: 10 in]
      n91 = Subtract(x=w153, y=w160) -> (x-y=w163:dbl)
      n92 = To Double Precision Float(number=w158) -> (double precision float=w156:dbl)
      n93 = Multiply(x=w163, y=1000.0) -> (x*y=w161:dbl)
      n94 = global write "VisionGlobal.vi" "Vision Count BR"(w158) -> ()
      n95 = call <vilib>:"AnalogDelay_Execute.vi"("Time"=w153, "Delay Time"=w159, "Input"=w156) -> ("Output"=w157:dbl)  [unwired: 7 in, 1 out]
      n96 = global write "VisionGlobal.vi" "Vision_BackRight_Latency_MS"(w161) -> ()
      n97 = global write "VisionGlobal.vi" "Vision_BackRightTime_Sec"(w160) -> ()
      n98 = global write "VisionGlobal.vi" "Vision_BackRightAng_Deg"(w164) -> ()
      n99 = global write "VisionGlobal.vi" "Vision_BackRightX_Ft"(w166) -> ()
      n100 = global write "VisionGlobal.vi" "Vision_BackRightY_Ft"(w165) -> ()
      n101 = Subtract(x=w156, y=w157) -> (x-y=w155:dbl)
      n102 = To Long Integer(number=w155) -> (32bit integer=w154:i32)
      n103 = global write "VisionGlobal.vi" "Vision_BackRight_LastSecCount"(w154) -> ()
    }
  }
  n104 = case shown="True" w9 {
    tunnel: w6 -> [_ w189]
    tunnel: w4 -> [_ w179]
    tunnel: w15 -> [_ w172]
    frame False {
    }
    frame True {
      w178 = 1.0  # Delay Time Seconds
      # "Delay"
      n105 = global read "VisionGlobal.vi" "Vision Count BB"() -> (w190:i32)
      n106 = call <vilib>:"Pose2d_getXYAngle.vi"("in POSE"=w189) -> ("Angle"=w186:dbl, "Y"=w187:dbl, "X"=w188:dbl)  [unwired: 8 in]
      n107 = Increment(x=w190) -> (x+1=w177:i32)
      n108 = call <vilib>:"Conv_Meters_Feet.vi"("Meters"=w187) -> ("Feet"=w184:dbl)  [unwired: 10 in]
      n109 = call <vilib>:"Conv_Radians_Deg.vi"("Radians"=w186) -> ("Degrees"=w183:dbl)  [unwired: 10 in]
      n110 = call <vilib>:"Conv_Meters_Feet.vi"("Meters"=w188) -> ("Feet"=w185:dbl)  [unwired: 10 in]
      n111 = Subtract(x=w172, y=w179) -> (x-y=w182:dbl)
      n112 = To Double Precision Float(number=w177) -> (double precision float=w175:dbl)
      n113 = Multiply(x=w182, y=1000.0) -> (x*y=w180:dbl)
      n114 = global write "VisionGlobal.vi" "Vision Count BB"(w177) -> ()
      n115 = call <vilib>:"AnalogDelay_Execute.vi"("Time"=w172, "Delay Time"=w178, "Input"=w175) -> ("Output"=w176:dbl)  [unwired: 7 in, 1 out]
      n116 = global write "VisionGlobal.vi" "Vision_BackBack_Latency_MS"(w180) -> ()
      n117 = global write "VisionGlobal.vi" "Vision_BackBackTime_Sec"(w179) -> ()
      n118 = global write "VisionGlobal.vi" "Vision_BackBackAng_Deg"(w183) -> ()
      n119 = global write "VisionGlobal.vi" "Vision_BackBackX_Ft"(w185) -> ()
      n120 = global write "VisionGlobal.vi" "Vision_BackBackY_Ft"(w184) -> ()
      n121 = Subtract(x=w175, y=w176) -> (x-y=w174:dbl)
      n122 = To Long Integer(number=w174) -> (32bit integer=w173:i32)
      n123 = global write "VisionGlobal.vi" "Vision_BackBack_LastSecCount"(w173) -> ()
    }
  }
  n124 = call "DriveGetYawRaw.vi"() -> ("YawRaw"=w91:dbl)  [unwired: 11 in]
  n125 = case shown="True" w107 {
    tunnel: w86 -> [_ w208]
    tunnel: w84 -> [_ w198]
    tunnel: w15 -> [_ w191]
    frame False {
    }
    frame True {
      w197 = 1.0  # Delay Time Seconds
      # "Delay"
      n126 = global read "VisionGlobal.vi" "Vision Count L"() -> (w209:i32)
      n127 = call <vilib>:"Pose2d_getXYAngle.vi"("in POSE"=w208) -> ("Angle"=w205:dbl, "Y"=w206:dbl, "X"=w207:dbl)  [unwired: 8 in]
      n128 = Increment(x=w209) -> (x+1=w196:i32)
      n129 = call <vilib>:"Conv_Meters_Feet.vi"("Meters"=w206) -> ("Feet"=w203:dbl)  [unwired: 10 in]
      n130 = call <vilib>:"Conv_Radians_Deg.vi"("Radians"=w205) -> ("Degrees"=w202:dbl)  [unwired: 10 in]
      n131 = call <vilib>:"Conv_Meters_Feet.vi"("Meters"=w207) -> ("Feet"=w204:dbl)  [unwired: 10 in]
      n132 = Subtract(x=w191, y=w198) -> (x-y=w201:dbl)
      n133 = To Double Precision Float(number=w196) -> (double precision float=w194:dbl)
      n134 = Multiply(x=w201, y=1000.0) -> (x*y=w199:dbl)
      n135 = global write "VisionGlobal.vi" "Vision Count L"(w196) -> ()
      n136 = call <vilib>:"AnalogDelay_Execute.vi"("Time"=w191, "Delay Time"=w197, "Input"=w194) -> ("Output"=w195:dbl)  [unwired: 7 in, 1 out]
      n137 = global write "VisionGlobal.vi" "Vision_Left_Latency_MS"(w199) -> ()
      n138 = global write "VisionGlobal.vi" "Vision_LeftTime_Sec"(w198) -> ()
      n139 = Subtract(x=w194, y=w195) -> (x-y=w193:dbl)
      n140 = global write "VisionGlobal.vi" "Vision_LeftAng_Deg"(w202) -> ()
      n141 = global write "VisionGlobal.vi" "Vision_LeftX_Ft"(w204) -> ()
      n142 = global write "VisionGlobal.vi" "Vision_LeftY_Ft"(w203) -> ()
      n143 = To Long Integer(number=w193) -> (32bit integer=w192:i32)
      n144 = global write "VisionGlobal.vi" "Vision_Left_LastSecCount"(w192) -> ()
    }
  }
  n145 = call <vilib>:"DigSeqLogic_One_Shot.vi"("Time"=w15, "OneShot"=w78, "Input"=w77) -> ("Output"=w76:bool)  [unwired: 7 in, 1 out]
  n146 = case shown="True" w108 {
    tunnel: w85 -> [_ w227]
    tunnel: w83 -> [_ w220]
    tunnel: w15 -> [_ w210]
    frame False {
    }
    frame True {
      w216 = 1.0  # Delay Time Seconds
      # "Delay"
      n147 = call <vilib>:"Pose2d_getXYAngle.vi"("in POSE"=w227) -> ("Angle"=w224:dbl, "Y"=w225:dbl, "X"=w226:dbl)  [unwired: 8 in]
      n148 = global read "VisionGlobal.vi" "Vision Count R"() -> (w228:i32)
      n149 = call <vilib>:"Conv_Meters_Feet.vi"("Meters"=w226) -> ("Feet"=w223:dbl)  [unwired: 10 in]
      n150 = call <vilib>:"Conv_Radians_Deg.vi"("Radians"=w224) -> ("Degrees"=w221:dbl)  [unwired: 10 in]
      n151 = Subtract(x=w210, y=w220) -> (x-y=w219:dbl)
      n152 = Multiply(x=w219, y=1000.0) -> (x*y=w217:dbl)
      n153 = call <vilib>:"Conv_Meters_Feet.vi"("Meters"=w225) -> ("Feet"=w222:dbl)  [unwired: 10 in]
      n154 = Increment(x=w228) -> (x+1=w212:i32)
      n155 = To Double Precision Float(number=w212) -> (double precision float=w214:dbl)
      n156 = call <vilib>:"AnalogDelay_Execute.vi"("Time"=w210, "Delay Time"=w216, "Input"=w214) -> ("Output"=w215:dbl)  [unwired: 7 in, 1 out]
      n157 = Subtract(x=w214, y=w215) -> (x-y=w213:dbl)
      n158 = global write "VisionGlobal.vi" "Vision_Right_Latency_MS"(w217) -> ()
      n159 = global write "VisionGlobal.vi" "Vision_RightTime_Sec"(w220) -> ()
      n160 = global write "VisionGlobal.vi" "Vision_RightAng_Deg"(w221) -> ()
      n161 = global write "VisionGlobal.vi" "Vision_RightX_Ft"(w223) -> ()
      n162 = global write "VisionGlobal.vi" "Vision_RightY_Ft"(w222) -> ()
      n163 = global write "VisionGlobal.vi" "Vision Count R"(w212) -> ()
      n164 = To Long Integer(number=w213) -> (32bit integer=w211:i32)
      n165 = global write "VisionGlobal.vi" "Vision_Right_LastSecCount"(w211) -> ()
    }
  }
  n166 = Boolean To (0,1)(Boolean=w108) -> (0, 1=w103:i16)
  n167 = Boolean To (0,1)(Boolean=w107) -> (0, 1=w106:i16)
  n168 = Not(x=w76) -> (.not. x?=w75:bool)
  n169 = call "DriveGetSwerveKinematics.vi"() -> ("SWERVE_DRIVE_KINEMATICS"=w88:T20)  [unwired: 11 in]
  n170 = Boolean To (0,1)(Boolean=w10) -> (0, 1=w11:i16)
  n171 = Boolean To (0,1)(Boolean=w9) -> (0, 1=w14:i16)
  n172 = Multiply(x=w106, y=i16 2) -> (x*y=w104:i16)
  n173 = Unbundle By Name(w88) -> ("Modules"=w87:T18[])
  n174 = Multiply(x=w14, y=i16 2) -> (x*y=w12:i16)
  n175 = call "DriveGetModulePositions.vi"() -> ("Swerve_Drive_Modual_Positions"=w92:T23[])  [unwired: 11 in]
  n176 = call <vilib>:"SwerveDrivePoseEst2_Pack_Config.vi"("Wheel_Locations M"=w87, "Vision Heading std dev Rad"=w101, "Odom X std dev M"=w100, "Vision Y std dev M"=w99, "Vision X std dev M"=w98, "Odom Heading std dev Rad"=w97, "Odom Y std dev M"=w96) -> ("SwervePoseEst2Config"=w95:T24)  [unwired: 4 in]
  n177 = call "VisionGetInitialAbsPose.vi"() -> ("InitialABSPose"=w81:T17)  [unwired: 10 in]
  n178 = Add(x=w103, y=w104) -> (x+y=w102:i16)
  n179 = Add(x=w11, y=w12) -> (x+y=w8:i16)
  n180 = global write "VisionGlobal.vi" "VisionFPGATime"(w15) -> ()
  n181 = case shown="3" w8 {
    tunnel: w7 -> [_ w233 _ w244]
    tunnel: w6 -> [_ _ w236 w243]
    tunnel: [FALSE ("Found") TRUE ("Found") TRUE ("Found") TRUE ("Found")] -> w2
    tunnel: w5 -> [_ w234 _ w241]
    tunnel: w4 -> [_ _ w237 w240]
    tunnel: [T17 {"TRANSLATION"={"X"=0.0, "Y"=0.0}, "ROTATION"={"VALUE"=0.0, "COS"=1.0, "SIN"=0.0}} ("Nearest Pose") w233 w236 w245] -> w3
    tunnel: [0.0 w234 w237 w239] -> w1
    frame 0, Default {
      # "None :((((("
    }
    frame 1 {
      # "Top (back right) camera"
    }
    frame 2 {
      # "Bottom (back back) camera"
    }
    frame 3 {
      # "Now it does average...\nby interpolation..."
      # "pick one \n(the one closest to robot)"
      # "Bothish (closest to robot)"
      n182 = call <vilib>:"Pose2d_Interpolate.vi"("T"=0.5, "EndValue Pose"=w243, "in POSE"=w244) -> ("Interpolated Pose"=w245:T17)  [unwired: 8 in]
      n183 = Max & Min(x=w241, y=w240) -> (max(x,y)=w239:dbl)  [unwired: 1 out]
    }
  }
  n184 = case shown="0, Default" w102 {
    tunnel: w85 -> [_ w250 _ w261]
    tunnel: w86 -> [_ _ w253 w260]
    tunnel: [w247 TRUE ("Found") TRUE ("Found") TRUE ("Found")] -> w82
    tunnel: w83 -> [_ w251 _ w258]
    tunnel: w84 -> [_ _ w254 w257]
    tunnel: [w248 w250 w253 w262] -> w90
    tunnel: [w246 w251 w254 w256] -> w89
    tunnel: w3 -> [w248 _ _ _]
    tunnel: w2 -> [w247 _ _ _]
    tunnel: w1 -> [w246 _ _ _]
    frame 0, Default {
      # "None :((((("
    }
    frame 1 {
      # "Top (right) camera"
    }
    frame 2 {
      # "Bottom (left) camera"
    }
    frame 3 {
      # "Now it does average...\nby interpolation..."
      # "pick one \n(the one closest to robot)"
      # "Bothish (closest to robot)"
      n185 = call <vilib>:"Pose2d_Interpolate.vi"("T"=0.5, "EndValue Pose"=w260, "in POSE"=w261) -> ("Interpolated Pose"=w262:T17)  [unwired: 8 in]
      n186 = Max & Min(x=w258, y=w257) -> (max(x,y)=w256:dbl)  [unwired: 1 out]
    }
  }
  n187 = call <vilib>:"SwerveDrivePoseEst2_Execute.vi"("Vision TImeStamp_Seconds"=w89, "SwervePoseEst2Config"=w95, "visionRobotPose"=w90, "Game Started"=w75, "Add Vision Meas"=w82, "InitialPose"=w81, "Pass Through Time"=w15, "Gyro Degrees"=w91, "Module Positions"=w92) -> ("Error"=w93:bool, "Estimated Pose"=w94:T17)  [unwired: 1 in]
  n188 = feedback-in #1(w94) -> ()
  n189 = global write "VisionGlobal.vi" "Odom Error"(w93) -> ()
  n190 = call "VisionSetCurrentAbsPose.vi"("Current ABS Pose"=w94) -> ()  [unwired: 11 in]
  "error out" <- "error in (no error)"
